vi "Get SMO PGSQL Log Paths.vi"(5 "getAll Cluster":variant, 7 "Default Paths":string, 8 "error in (no error)":errorcluster, 11 "Instrument.FrameworkTemplate":refnum<class "Instrument.Temperhum.lvclass">) -> (0 "error out":errorcluster, 2 "Paths":string, 3 "Instrument.FrameworkTemplate out":refnum<class "Instrument.Temperhum.lvclass">)   [LabVIEW 2019, in "Instrument.Temperhum.lvclass"]
uses:
  Instrument.Temperhum.lvclass
  Typedefs/Instrument.Temperhum.getAll--Cluster.ctl
  <userlib>/LevyLab/LV-Data/LV-Data.PG/LV-Data.PGSQL.lvclass
  <userlib>/LevyLab/LV-Data/LV-Data.PG/API/Write Variable (one-row).vi
  <userlib>/LevyLab/Instrument Framework/Instrument Types/VSource/Instrument.VSource.lvclass
  <vilib>/JKI/JKI SMO/SMO/SMO.lvclass
  C:/Program Files (x86)/National Instruments/LabVIEW 2019/user.lib/LevyLab/Instrument Framework/Instrument Types/VSource/Instrument.VSource.lvclass
  C:/Program Files (x86)/National Instruments/LabVIEW 2019/user.lib/LevyLab/Instrument Framework/SMOs/Instrument/Instrument.lvclass
  C:/Program Files (x86)/National Instruments/LabVIEW 2019/vi.lib/JKI/JKI SMO/SMO/SMO.lvclass
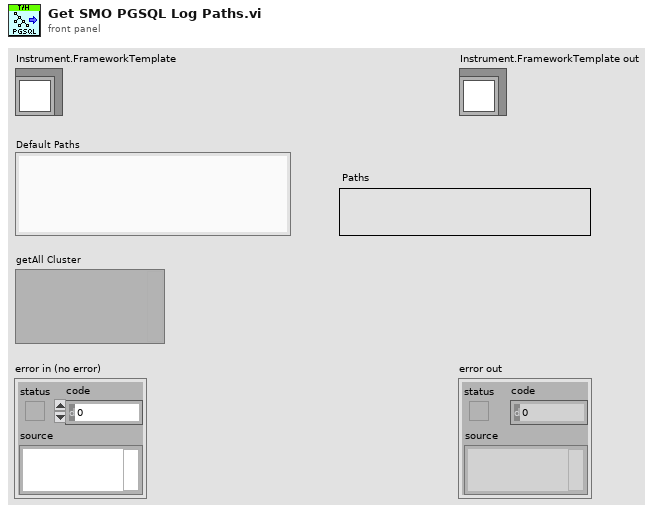
[diagram p1: front panel]
types:
  T1 = typedef "Instrument.Temperhum.lvclass/Instrument.Temperhum.getAll--Cluster.ctl" = cluster{"Temperature (K)":dbl, "Humidity (%RH)":dbl}
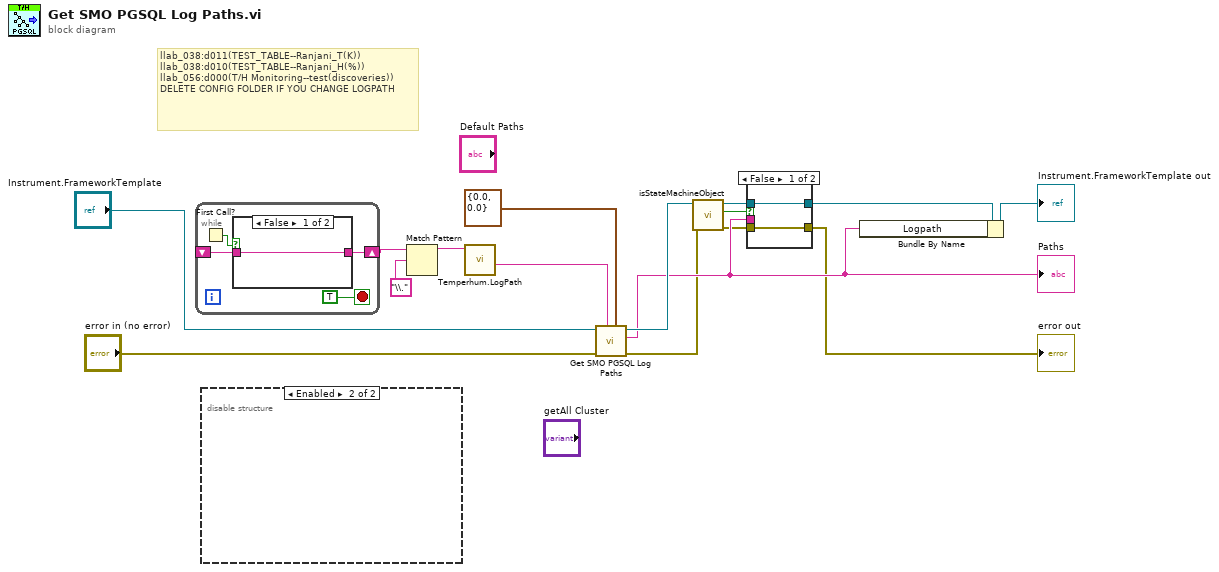
[diagram p0: block diagram]
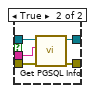
[diagram p2: hidden frame]
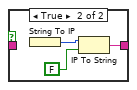
[diagram p3: hidden frame]
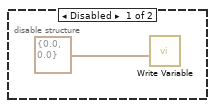
[diagram p4: hidden frame]
diagram:
  # "llab_038:d011(TEST_TABLE--Ranjani_T(K))\nllab_038:d010(TEST_TABLE--Ranjani_H(%))\nllab_056:d000(T/H Monitoring--test(discoveries))\nDELETE CONFIG FOLDER IF YOU CHANGE LOGPATH"
  n1 = while {
    shift-right: [w20] -> w11
    shift-left: _ -> [w17]
    stop <- TRUE stop-if-true
    n2 = First Call?() -> (First Call?: T/F=w18:bool)
    n3 = case shown="False" w18 {
      tunnel: [w21 w22] -> w20
      tunnel: w17 -> [w21 _]
      frame False {
      }
      frame True {
        n4 = String To IP() -> (0:w23:u32)  [unwired: 1 in]
        n5 = IP To String(1:FALSE, 2:w23) -> (0:w22:string)
      }
    }
  }
  n6 = disable-structure shown="Enabled" {
    frame Disabled {
      n7 = call-poly <userlib>:"Write Variable.vi"("Data"=T1 {"Temperature (K)"=0.0, "Humidity (%RH)"=0.0} ("getAll")) -> ()  [unwired: 7 in, 4 out]
    }
    frame Enabled {
    }
  }
  n8 = Match Pattern(string=w11, regular expression="\\.") -> (before substring=w12:string)  [unwired: 1 in, 3 out]
  n9 = call "Temperhum.LogPath.vi"("Computer Name"=w12) -> ("Paths"=w8:string)  [unwired: 9 in]
  n10 = call-parent "Get SMO PGSQL Log Paths.vi"("getAll Cluster"=T1 {"Temperature (K)"=0.0, "Humidity (%RH)"=0.0} ("getAll"), "Default Paths"=w8, "error in (no error)"="error in (no error)", "Instrument in"="Instrument.FrameworkTemplate") -> ("error out"=w5:errorcluster, "Paths"=w6:string, "Instrument out"=w7:refnum<class "Instrument.Temperhum.lvclass">)  [unwired: 5 in]
  "Paths" <- w6
  n11 = call <vilib>:"isStateMachineObject.vi"("error in (no error)"=w5, "SMO"=w7) -> ("error out"=w4:errorcluster, "is SMO?"=w3:bool, "SMO out"=w2:refnum<class "Instrument.Temperhum.lvclass">)  [unwired: 7 in]
  n12 = case shown="False" w3 {
    tunnel: [w26 w32] -> w9
    tunnel: [w27 w31] -> w1
    tunnel: w2 -> [w26 w30]
    tunnel: w6 -> [_ w28]
    tunnel: w4 -> [w27 w29]
    frame False {
    }
    frame True {
      n13 = call "Get PGSQL Info.vi"("error in (no error)"=w29, "Get PGSQL Info"=w28, "Instrument.Temperhum in"=w30) -> ("error out"=w31:errorcluster, "Instrument.Temperhum out"=w32:refnum<class "Instrument.Temperhum.lvclass">)  [unwired: 7 in]
    }
  }
  "error out" <- w1
  n14 = Bundle By Name(cluster=w9, "Logpath"=w6) -> (→"Instrument.FrameworkTemplate out":refnum<class "Instrument.Temperhum.lvclass">)
